vi "get_subcomponents.vi"(8 "error in (no error)":errorcluster, 11 "ScanHeadDL090202 in":refnum<class "ScanHeadDL090202.lvclass">) -> (0 "error out":errorcluster, 2 "subcomponents":T1[](array[typedef]), 3 "ScanHeadDL090202 out":refnum<class "ScanHeadDL090202.lvclass">)   [LabVIEW 2010, in "ScanHeadDL090202.lvclass"]
uses:
  ScanHeadDL090202.lvclass
  common/classes/GenericComponent/GenericComponent/subcomponent_cluster.ctl
  common/classes/GenericComponent/GenericComponent/GenericComponent.lvclass
  ScanHeadDL090202.lvclass/ScanHeadDL090202.ctl
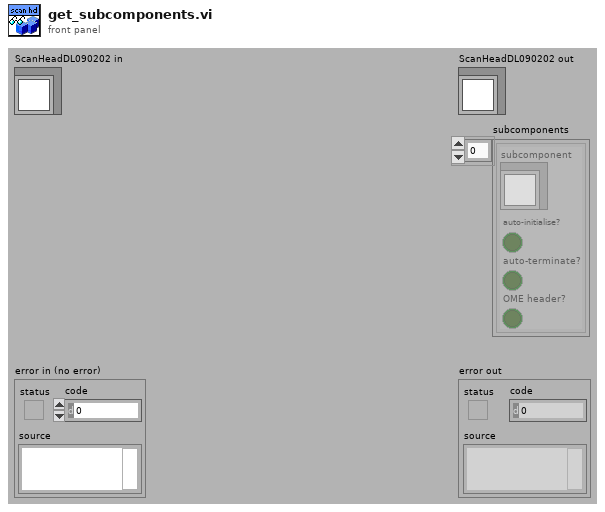
[diagram p1: front panel]
types:
  T1 = typedef "GenericComponent.lvclass/subcomponent_cluster.ctl" = cluster{"subcomponent":refnum<class "GenericComponent.lvclass">, "auto-initialise?":bool, "auto-terminate?":bool, "OME header?":bool}
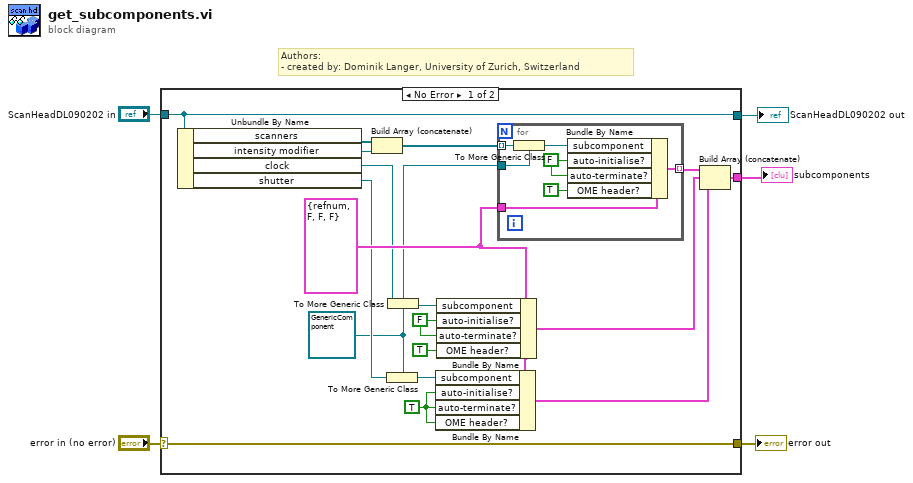
[diagram p0: block diagram]
diagram:
  # "Authors: \n- created by: Dominik Langer, University of Zurich, Switzerland"
  n1 = case shown="No Error" "error in (no error)" {
    selector: "error in (no error)" -> [w21 w31]
    tunnel: "ScanHeadDL090202 in" -> [w23 w32]
    tunnel: [w23 w32] -> w3
    tunnel: [w22 _] -> w1
    tunnel: [w21 w31] -> w2
    frame No Error {
      w6 = refnum<class "GenericComponent.lvclass"> refnum ("subcomponent")
      w11 = FALSE
      w12 = TRUE
      w16 = T1 {"subcomponent"=refnum, "auto-initialise?"=FALSE, "auto-terminate?"=FALSE, "OME header?"=FALSE} ("subcomponent cluster")
      n2 = Unbundle By Name(w23) -> ("scanners"=w19:refnum<class "GenericSignalWriter.lvclass">[], "intensity modifier"=w20:refnum<class "GenericSignalWriter.lvclass">, "clock"=w10:refnum<class "GenericClock.lvclass">, "shutter"=w8:refnum<class "GenericShutter.lvclass">)
      n3 = Build Array (concatenate)(w19, w20) -> (w18:refnum<class "GenericSignalWriter.lvclass">[])
      n4 = To More Generic Class(target class=w6, reference=w8) -> (generic class reference=w7:refnum<class "GenericComponent.lvclass">)
      n5 = To More Generic Class(target class=w6, reference=w10) -> (generic class reference=w9:refnum<class "GenericComponent.lvclass">)
      n6 = Bundle By Name(cluster=w16, "subcomponent"=w7, "auto-initialise?"=w12, "auto-terminate?"=w12, "OME header?"=w12) -> (w14:T1)
      n7 = Bundle By Name(cluster=w16, "subcomponent"=w9, "auto-initialise?"=w11, "auto-terminate?"=w11, "OME header?"=TRUE) -> (w15:T1)
      n8 = for {
        tunnel: w18 -> [w28] mode=indexing
        tunnel: w16 -> [w30]
        tunnel: [w29] -> w17 mode=indexing
        tunnel: w6 -> [w26]
        w25 = FALSE
        n9 = To More Generic Class(target class=w26, reference=w28) -> (generic class reference=w27:refnum<class "GenericComponent.lvclass">)
        n10 = Bundle By Name(cluster=w30, "subcomponent"=w27, "auto-initialise?"=w25, "auto-terminate?"=w25, "OME header?"=TRUE) -> (w29:T1)
      }
      n11 = Build Array (concatenate)(w17, w15, w14) -> (w22:T1[])
    }
    frame Error {
    }
  }
  "error out" <- w2
  "ScanHeadDL090202 out" <- w3
  "subcomponents" <- w1
